vi "removeQuotations.vi"(8 "error in (no error)":errorcluster, 10 "quoteIn":string, 11 "AttributeReader in":refnum<class "XMLAttributeParser.lvclass">) -> (0 "error out":errorcluster, 2 "quoteOut":string, 3 "AttributeReader out":refnum<class "XMLAttributeParser.lvclass">)   [LabVIEW 2016, in "XML.lvlib" / "XMLAttributeParser.lvclass"]
doc: "This method reoves quotations on the outside of the string by getting rid of the first and last character in the string."
uses:
  <userlib>/Common/XML/XMLAttributeParser/XMLAttributeParser.lvclass
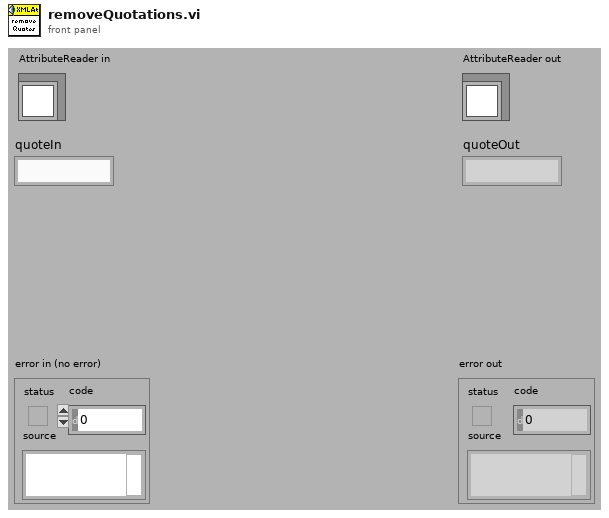
[diagram p1: front panel]
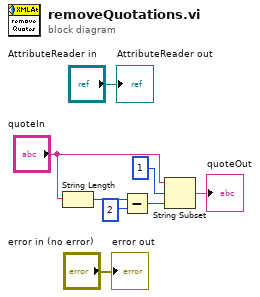
[diagram p0: block diagram]
diagram:
  n1 = String Length(string="quoteIn") -> (length=w3:i32)
  n2 = Subtract(x=w3, y=2) -> (x-y=w6:i32)
  n3 = String Subset(string="quoteIn", offset (0)=1, length (rest)=w6) -> (substring=→"quoteOut":string)
  "error out" <- "error in (no error)"
  "AttributeReader out" <- "AttributeReader in"
